vi "Autonomous Independent.vi"   [LabVIEW 2012]
doc: "This VI is called when autonomous begins, and will automatically be terminated when autonomous ends. You can carry out timed or sensor driven robot movement independently without needing to return to the caller."
uses:
  Robot Global Data.vi
  Globals/Useful Values.vi
  Globals/Shooter Elevation Positons.vi
panel:
  # "Be sure to right-click and choose Data Operations>>Make Current Value default if you want to save the array values with the VI"
types:
  T1 = typedef "WPI_DriverStationAllianceInfo.ctl" = enum16{"Red", "Blue", "Invalid"}
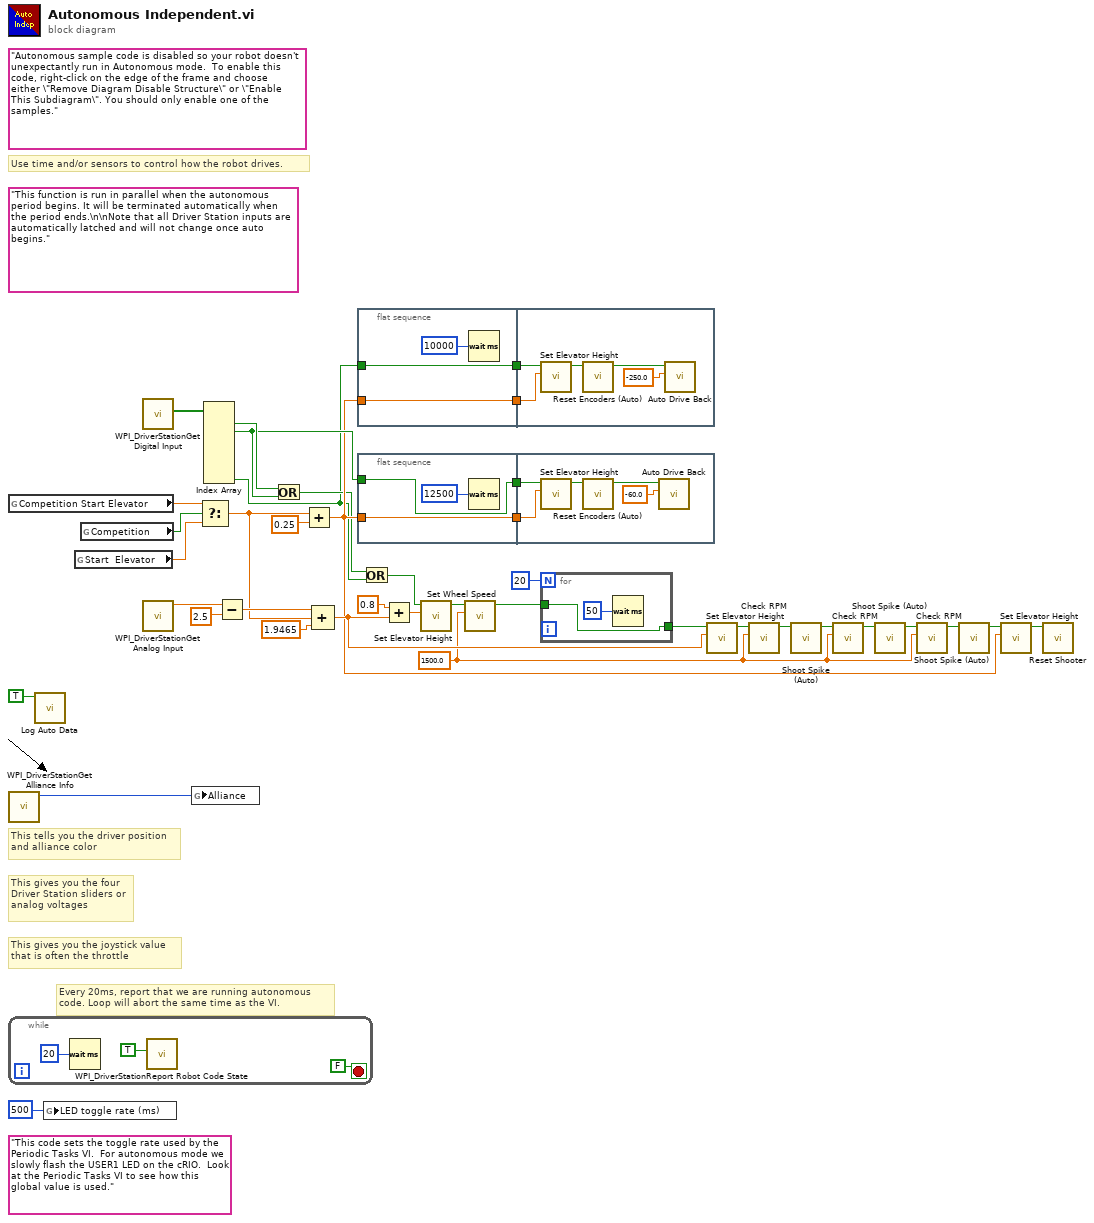
[diagram p0: block diagram]
diagram:
  w8 = 1500.0 ("RPM (1900)")
  (unwired) "This code sets the toggle rate used by the Periodic Tasks VI.  For autonomous mode we slowly flash the USER1 LED on the cRIO.  Look at the Periodic Tasks VI to see how this global value is used."
  (unwired) "Autonomous sample code is disabled so your robot doesn't unexpectantly run in Autonomous mode.  To enable this code, right-click on the edge of the frame and choose either \"Remove Diagram Disable Structure\" or \"Enable This Subdiagram\". You should only enable one of the samples."
  (unwired) "This function is run in parallel when the autonomous period begins. It will be terminated automatically when the period ends.\n\nNote that all Driver Station inputs are automatically latched and will not change once auto begins."
  # "Every 20ms, report that we are running autonomous\ncode. Loop will abort the same time as the VI."
  # "This gives you the joystick value\nthat is often the throttle"
  # "Use time and/or sensors to control how the robot drives."
  # "This tells you the driver position\nand alliance color"
  # "This gives you the four\nDriver Station sliders or\nanalog voltages"
  n1 = global read "Shooter Elevation Positons.vi" "Competition Start Elevator"() -> (w36:dbl)
  n2 = call <vilib>:"WPI_DriverStationGet Alliance Info.vi"() -> ("Alliance"=w21:T1)  [unwired: 11 out]
  n3 = while {
    stop <- FALSE stop-if-true
    n4 = Wait (ms)(milliseconds to wait=u32 20) -> ()  [unwired: 1 out]
    n5 = call <vilib>:"WPI_DriverStationReport Robot Code State.vi"("Autonomous"=TRUE) -> ()  [unwired: 10 in, 1 out]
  }
  n6 = call "Log Auto Data.vi"("Record"=TRUE) -> ()  [unwired: 10 in, 1 out]
  n7 = global write "Robot Global Data.vi" "LED toggle rate (ms)"(u32 500 ("LED ms toggle rate")) -> ()
  n8 = global read "Shooter Elevation Positons.vi" "Start  Elevator"() -> (w34:dbl)
  n9 = global read "Useful Values.vi" "Competition"() -> (w35:bool)
  n10 = call <vilib>:"WPI_DriverStationGet Digital Input.vi"() -> ("Driver Station Digital Input (1-8)"=w39:bool[])  [unwired: 11 out]
  n11 = call <vilib>:"WPI_DriverStationGet Analog Input.vi"() -> ("Analog 1 (V)"=w32:dbl)  [unwired: 11 out]
  n12 = global write "Useful Values.vi" "Alliance"(w21) -> ()
  n13 = Select(t=w36, s=w35, f=w34) -> (s? t:f=w29:dbl)
  n14 = Index Array(array=w39) -> (element #1=w37:bool, element #2=w26:bool, element #8=w1:bool)  [unwired: 8 in, 5 out]
  n15 = Subtract(x=w32, y=2.5) -> (x-y=w30:dbl)
  n16 = Or(x=w37, y=w26) -> (x .or. y?=w2:bool)
  n17 = Add(x=w29, y=0.25) -> (x+y=w4:dbl)
  n18 = Compound Arithmetic op=ADD(w30, w29, 1.9465 ("value")) -> (w17:dbl)
  n19 = flat-sequence {
    tunnel: w1 -> [w44]
    tunnel: [w44] -> w6
    tunnel: [w43] -> w5
    tunnel: w4 -> [w43]
    tunnel: w6 -> [w47]
    tunnel: w5 -> [w46]
    frame #0 {
      n20 = Wait (ms)(milliseconds to wait=u32 10000) -> ()  [unwired: 1 out]
    }
    frame #1 {
      n21 = call "Set Elevator Height.vi"("Height"=w46, "Execute?"=w47) -> ("Done"=w48:bool)  [unwired: 9 in]
      n22 = call "Reset Encoders (Auto).vi"("Execute?"=w48) -> ("Done"=w49:bool)  [unwired: 10 in]
      n23 = call "Auto Drive Back.vi"("Distance"=-250.0, "Execute?"=w49) -> ()  [unwired: 9 in, 1 out]
    }
  }
  n24 = flat-sequence {
    tunnel: w26 -> [w52]
    tunnel: [w52] -> w25
    tunnel: [w51] -> w24
    tunnel: w4 -> [w51]
    tunnel: w25 -> [w55]
    tunnel: w24 -> [w54]
    frame #0 {
      n25 = Wait (ms)(milliseconds to wait=u32 12500) -> ()  [unwired: 1 out]
    }
    frame #1 {
      n26 = call "Set Elevator Height.vi"("Height"=w54, "Execute?"=w55) -> ("Done"=w56:bool)  [unwired: 9 in]
      n27 = call "Reset Encoders (Auto).vi"("Execute?"=w56) -> ("Done"=w57:bool)  [unwired: 10 in]
      n28 = call "Auto Drive Back.vi"("Distance"=-60.0, "Execute?"=w57) -> ()  [unwired: 9 in, 1 out]
    }
  }
  n29 = Or(x=w2, y=w1) -> (x .or. y?=w3:bool)
  n30 = Add(x=0.8, y=w17) -> (x+y=w15:dbl)
  n31 = call "Set Elevator Height.vi"("Height"=w15, "Execute?"=w3) -> ("Done"=w14:bool)  [unwired: 9 in]
  n32 = call "Set Wheel Speed.vi"("RPM"=w8, "Execute?"=w14) -> ("Done"=w13:bool)  [unwired: 9 in]
  n33 = for {
    N: 20 -> [_]
    tunnel: w13 -> [w59]
    tunnel: [w59] -> w19
    n34 = Wait (ms)(milliseconds to wait=u32 50) -> ()  [unwired: 1 out]
  }
  n35 = call "Set Elevator Height.vi"("Height"=w17, "Execute?"=w19) -> ("Done"=w18:bool)  [unwired: 9 in]
  n36 = call "Check RPM.vi"("RPM Wanted"=w8, "Execute?"=w18) -> ("Done"=w27:bool)  [unwired: 9 in]
  n37 = call "Shoot Spike (Auto).vi"("Execute?"=w27) -> ("Done"=w12:bool)  [unwired: 10 in]
  n38 = call "Check RPM.vi"("RPM Wanted"=w8, "Execute?"=w12) -> ("Done"=w11:bool)  [unwired: 9 in]
  n39 = call "Shoot Spike (Auto).vi"("Execute?"=w11) -> ("Done"=w10:bool)  [unwired: 10 in]
  n40 = call "Check RPM.vi"("RPM Wanted"=w8, "Execute?"=w10) -> ("Done"=w9:bool)  [unwired: 9 in]
  n41 = call "Shoot Spike (Auto).vi"("Execute?"=w9) -> ("Done"=w23:bool)  [unwired: 10 in]
  n42 = call "Set Elevator Height.vi"("Height"=w4, "Execute?"=w23) -> ("Done"=w22:bool)  [unwired: 9 in]
  n43 = call "Reset Shooter.vi"("Execute?"=w22) -> ()  [unwired: 10 in, 1 out]
